vi "Sort rectangles from left to right.vi"(11 "Rectangles (Calibrated) IN":T1(array[cluster])) -> (3 "Rectangles (Calibrated) OUT":T1(array[cluster]))   [LabVIEW 2018]
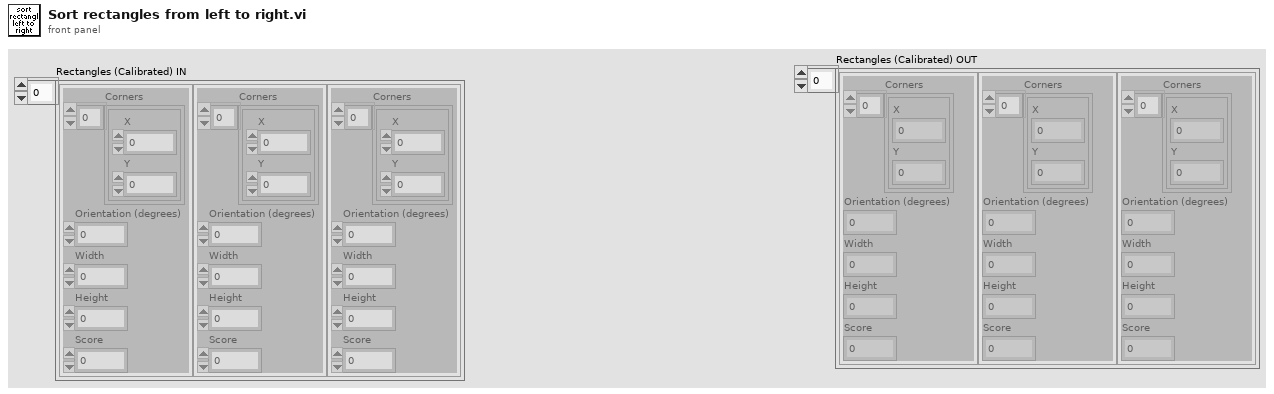
[diagram p1: front panel]
types:
  T1 = cluster{"Corners":cluster{"X":sgl, "Y":sgl}[], "Orientation (degrees)":dbl, "Width":dbl, "Height":dbl, "Score":dbl}[]
  T2 = cluster{"Corners":cluster{"X":sgl, "Y":sgl}[], "Orientation (degrees)":dbl, "Width":dbl, "Height":dbl, "Score":dbl}
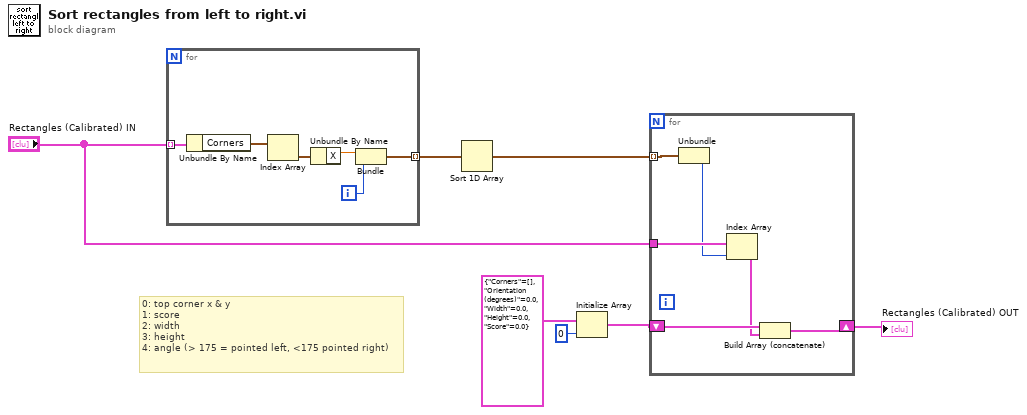
[diagram p0: block diagram]
diagram:
  # "0: top corner x & y\n1: score\n2: width\n3: height\n4: angle (> 175 = pointed left, <175 pointed right)"
  n1 = for {
    tunnel: "Rectangles (Calibrated) IN" -> [w13] mode=indexing
    tunnel: [w8] -> w5 mode=indexing
    i -> [w9]
    n2 = Unbundle By Name(w13) -> ("Corners"=w12:cluster{"X":sgl, "Y":sgl}[])
    n3 = Index Array(array=w12) -> (element=w11:cluster{"X":sgl, "Y":sgl})  [unwired: 1 in]
    n4 = Unbundle By Name(w11) -> ("X"=w10:sgl)
    n5 = Bundle("X"=w10, w9) -> (w8:cluster{"X":sgl, i32})  [unwired: 1 in]
  }
  n6 = Sort 1D Array(array=w5) -> (sorted array=w4:cluster{"X":sgl, i32}[])
  n7 = Initialize Array(T2 {"Corners"=[], "Orientation (degrees)"=0.0, "Width"=0.0, "Height"=0.0, "Score"=0.0} ("Rectangle Descriptor"), 0 ("dimension size")) -> (w3:T1)
  n8 = for {
    tunnel: w4 -> [w15] mode=indexing
    shift-right: [w16] -> w1
    shift-left: w3 -> [w19]
    tunnel: "Rectangles (Calibrated) IN" -> [w18]
    n9 = Unbundle(w15) -> (w14:i32)  [unwired: 1 out]
    n10 = Index Array(array=w18, index=w14) -> (element=w17:T2)
    n11 = Build Array (concatenate)(w19, w17) -> (w16:T1)
  }
  "Rectangles (Calibrated) OUT" <- w1
